vi "Build Data Frame.vi"(8 "error in (no error)":errorcluster, 9 "system info in":refnum<class "PMU System Info.lvclass">, 11 "measurement data":T1={"data valid? (T)"=TRUE, "PMU error? (F)"=FALSE, "PMU sync? (F)"=FALSE, "data sorting"=enum."by timestamp", "PMU trigger detected? (F)"=FALSE, "configuration changed? (F)"=FALSE, "df/dt [Hz/s]"=0.0, "analogs"=[], "digitals"=[], "frequency"=0.0, "phasors"=[], "reserved bits for security"=0, "trigger reason"=0, "timestamp"=timestamp(0 s since 1904-01-01), "time quality"=0, "unlocked time"=0} {"trigger reason" format="%04b"}) -> (0 "error out":errorcluster, 1 "system info out":refnum<class "PMU System Info.lvclass">, 3 "data frame":string)   [LabVIEW 2013, in "NI_EP_PMU.lvlib"]
doc: "LabVIEW no longer supports this VI. Use the Build Data Frame (Std 2011) VI instead.\n\nBuilds a data frame according to IEEE Std C37.118-2005."
uses:
  <vilib>/addons/Electrical Power/PMU/NI_EP_PMU.lvlib
  <vilib>/addons/Electrical Power/PMU/Common/Classes/PMU System Info/PMU System Info.lvclass
  <vilib>/addons/Electrical Power/PMU/Common/Controls/pmu_Measurement Data.ctl
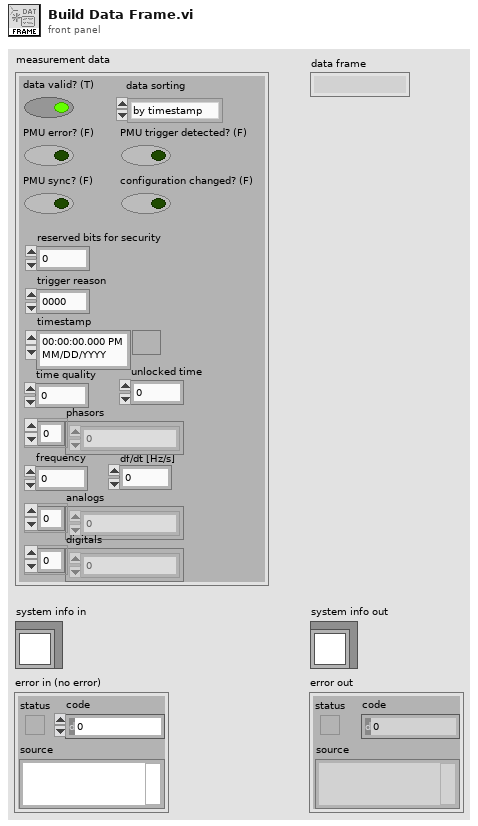
[diagram p1: front panel]
types:
  T1 = typedef "NI_EP_PMU.lvlib/pmu_Measurement Data.ctl" = cluster{"data valid? (T)":bool, "PMU error? (F)":bool, "PMU sync? (F)":bool, "data sorting":enum16{"by timestamp", "by arrival"}, "PMU trigger detected? (F)":bool, "configuration changed? (F)":bool, "df/dt [Hz/s]":sgl, "analogs":sgl[], "digitals":u16[], "frequency":sgl, "phasors":csg[], "reserved bits for security":u8, "trigger reason":u8, "timestamp":timestamp, "time quality":u8, "unlocked time":u32}
  T2 = typedef "NI_EP_PMU.lvlib/pmu_CFG Class.ctl" = cluster{"station name":string, "PMU ID":u16, "time base":u32, "nominal frequency":enum16{"50 Hz", "60 Hz"}, "reporting rate":i16, "phasor number":u16, "analog number":u16, "digital number":u16, "channel names":string[], "phasor units":u32[], "analog units":u32[], "digital units":u32[], "data format":u16, "number of PMUs":u16}
  T3 = typedef "LVDateTimeRec.ctl" = cluster{"fractional second":dbl, "second":i32, "minute":i32, "hour":i32, "day of month":i32, "month":i32, "year":i32, "day of week":i32, "day of year":i32, "DST":i32}
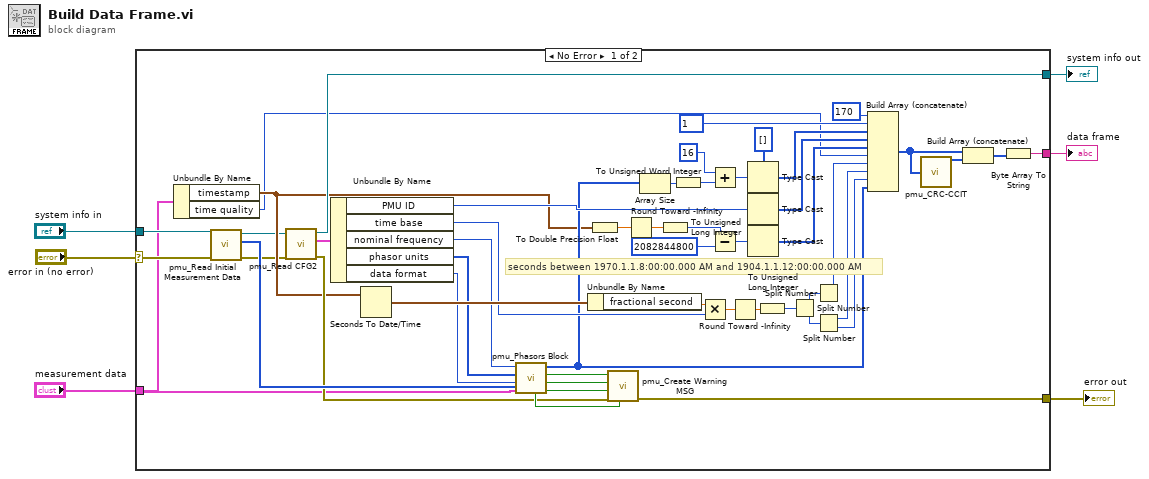
[diagram p0: block diagram]
diagram:
  n1 = case shown="No Error" "error in (no error)" {
    selector: "error in (no error)" -> [w25 w58]
    tunnel: [w57 _] -> w6
    tunnel: "system info in" -> [w26 w59]
    tunnel: "measurement data" -> [w12 _]
    tunnel: [w28 w59] -> w2
    tunnel: [w13 w58] -> w1
    frame No Error {
      w52 = u8[] [] ("appended array")
      # "seconds between 1970.1.1.8:00:00.000 AM and 1904.1.1.12:00:00.000 AM"
      n2 = Unbundle By Name(w12) -> ("timestamp"=w11:timestamp, "time quality"=w10:u8)
      n3 = call <vilib>:"pmu_Read Initial Measurement Data.vi"("error in (no error)"=w25, "system info in"=w26) -> ("error out"=w8:errorcluster, "init meas data"=w19:u8[], "system info out"=w9:refnum<class "PMU System Info.lvclass">)  [unwired: 7 in]
      n4 = call <vilib>:"pmu_Read CFG2.vi"("error in (no error)"=w8, "system info in"=w9) -> ("error out"=w14:errorcluster, "CFG-2"=w33:T2, "system info out"=w28:refnum<class "PMU System Info.lvclass">)  [unwired: 7 in]
      n5 = Unbundle By Name(w33) -> ("PMU ID"=w31:u16, "time base"=w32:u32, "nominal frequency"=w7:enum16{"50 Hz", "60 Hz"}, "phasor units"=w30:u32[], "data format"=w24:u16)
      n6 = Seconds To Date/Time(time stamp (now)=w11) -> (date time rec=w54:T3)  [unwired: 1 in]
      n7 = call <vilib>:"pmu_Phasors Block.vi"("init meas data"=w19, "measurement data"=w12, "data format"=w24, "phasor units"=w30, "nominal frequency"=w7) -> ("df/dt out of range"=w16:bool, "freq out of range"=w17:bool, "phasor out of range"=w18:bool, "data block"=w29:u8[], "analog out of range"=w15:bool)  [unwired: 2 in]
      n8 = Unbundle By Name(w54) -> ("fractional second"=w56:dbl)
      n9 = To Double Precision Float(number=w11) -> (double precision float=w23:dbl)
      n10 = call <vilib>:"pmu_Create Warning MSG.vi"("analog out of range"=w15, "error in (no error)"=w14, "df/dt out of range"=w16, "freq out of range"=w17, "phasor out of range"=w18) -> ("error out"=w13:errorcluster)  [unwired: 6 in]
      n11 = Round Toward -Infinity(1:w23) -> (0:w22:dbl)
      n12 = Array Size(array=w29) -> (size(s)=w36:i32)
      n13 = To Unsigned Long Integer(number=w22) -> (unsigned 32bit integer=w55:u32)
      n14 = To Unsigned Word Integer(number=w36) -> (unsigned 16bit integer=w38:u16)
      n15 = Multiply(x=w56, y=w32) -> (x*y=w20:dbl)
      n16 = Add(x=u16 16 ("y"), y=w38) -> (x+y=w47:u16)
      n17 = Subtract(x=w55, y=u32 2082844800 ("unsigned 32bit integer")) -> (x-y=w50:u32)
      n18 = Round Toward -Infinity(1:w20) -> (0:w21:dbl)
      n19 = Type Cast(type=w52, x=w47) -> (*(type *) &x=w48:u8[])
      n20 = Type Cast(type=w52, x=w31) -> (*(type *) &x=w49:u8[])
      n21 = Type Cast(type=w52, x=w50) -> (*(type *) &x=w51:u8[])
      n22 = To Unsigned Long Integer(number=w21) -> (unsigned 32bit integer=w53:u32)
      n23 = Split Number(x=w53) -> (hi(x)=w41:u16, lo(x)=w40:u16)
      n24 = Split Number(x=w41) -> (lo(x)=w42:u8)  [unwired: 1 out]
      n25 = Split Number(x=w40) -> (hi(x)=w43:u8, lo(x)=w44:u8)
      n26 = Build Array (concatenate)(u8 170 ("element"), u8 1 ("element"), w48, w49, w51, w10, w42, w43, w44, w29) -> (w45:u8[])
      n27 = call <vilib>:"pmu_CRC-CCIT.vi"("byte array"=w45) -> ("CRCbytes"=w46:u8[])  [unwired: 13 in, 1 out]
      n28 = Build Array (concatenate)(w45, w46) -> (w34:u8[])
      n29 = Byte Array To String(unsigned byte array=w34) -> (string=w57:string)
    }
    frame Error {
    }
  }
  "data frame" <- w6
  "error out" <- w1
  "system info out" <- w2
